vi "laba5.vi"() -> ()   [LabVIEW 2018]
uses:
  <vilib>/Utility/file.llb/Read Delimited Spreadsheet (DBL).vi
  <vilib>/Utility/file.llb/Write Delimited Spreadsheet (DBL).vi
panel:
  in  "File Path Control 2":path
  in  "File Path Control":path
  out "XY Graph":cluster{"all rows":dbl[], "all rows":dbl[]}[](graph)
  out "Waveform Graph 2":cluster{i32, i32, "all rows":dbl[]}(graph)
  out "Waveform Graph":cluster{i32, i32, "all rows":dbl[]}(graph)
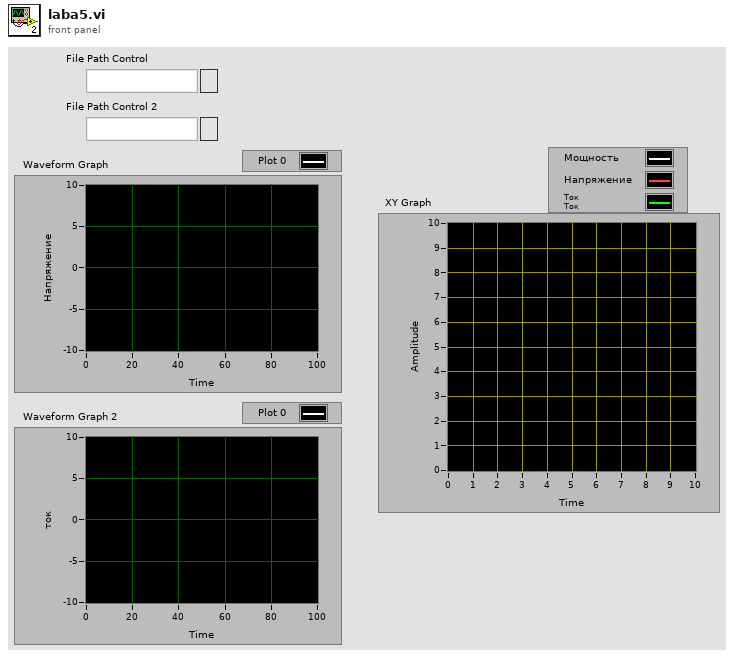
[diagram p1: front panel]
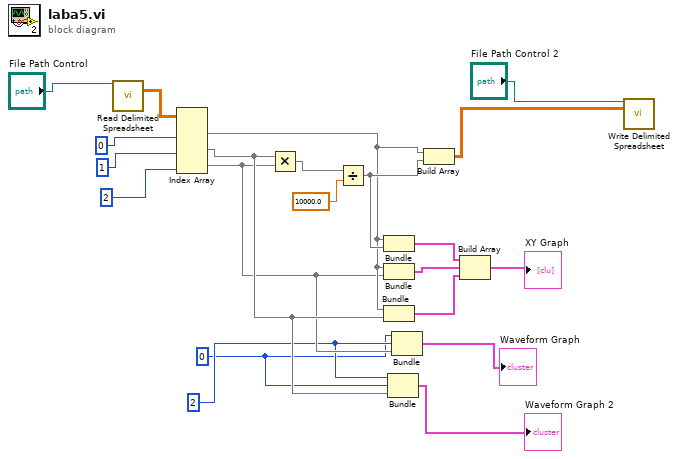
[diagram p0: block diagram]
diagram:
  w3 = 2
  w2 = 0
  n1 = call-poly <vilib>:"Read Delimited Spreadsheet.vi"("file path (dialog if empty)"="File Path Control") -> ("all rows"=w20:dbl[][])  [unwired: 9 in, 5 out]
  n2 = Index Array(array=w20, index (col) #1=0, index (col) #2=1, index (col) #3=2) -> (element #1=w10:dbl[], element #2=w6:dbl[], element #3=w5:dbl[])  [unwired: 3 in]
  n3 = Multiply(x=w6, y=w5) -> (x*y=w16:dbl[])
  n4 = Divide(x=w16, y=10000.0) -> (x/y=w14:dbl[])
  n5 = Bundle("all rows"=w10, w14) -> (w13:cluster{"all rows":dbl[], dbl[]})  [unwired: 1 in]
  n6 = Bundle("all rows"=w10, "all rows"=w5) -> (w9:cluster{"all rows":dbl[], "all rows":dbl[]})  [unwired: 1 in]
  n7 = Bundle("all rows"=w10, "all rows"=w6) -> (w8:cluster{"all rows":dbl[], "all rows":dbl[]})  [unwired: 1 in]
  n8 = Bundle(w3, w2, "all rows"=w6) -> (→"Waveform Graph 2":cluster{i32, i32, "all rows":dbl[]})  [unwired: 1 in]
  n9 = Bundle(w2, w3, "all rows"=w5) -> (→"Waveform Graph":cluster{i32, i32, "all rows":dbl[]})  [unwired: 1 in]
  n10 = Build Array(w10, w14) -> (w11:dbl[][])
  n11 = Build Array(w13, w9, w8) -> (→"XY Graph":cluster{"all rows":dbl[], "all rows":dbl[]}[])
  n12 = call-poly <vilib>:"Write Delimited Spreadsheet.vi"("file path (dialog if empty)"="File Path Control 2", "2D data"=w11) -> ()  [unwired: 12 in, 2 out]
